vi "Outcounter.vi"(11 "in control band":bool) -> ()   [LabVIEW 2019]
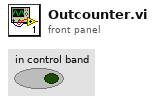
[diagram p1: front panel]
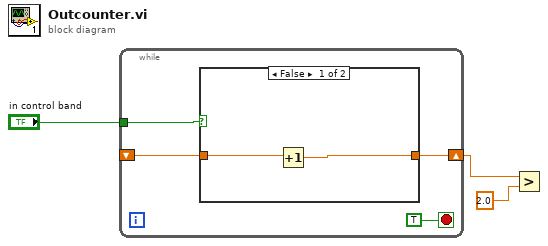
[diagram p0: block diagram]
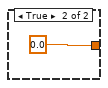
[diagram p2: hidden frame]
diagram:
  n1 = while {
    tunnel: "in control band" -> [w7]
    shift-right: [w6] -> w2
    shift-left: _ -> [w5]
    stop <- TRUE stop-if-true
    n2 = case shown="False" w7 {
      tunnel: [w9 0.0] -> w6
      tunnel: w5 -> [w8 _]
      frame False {
        n3 = Increment(x=w8) -> (x+1=w9:dbl)
      }
      frame True {
      }
    }
  }
  n4 = Greater?(x=w2, y=2.0) -> ()  [unwired: 1 out]
